vi "Display Hardware Error.vi"(8 "error in (no error)":errorcluster) -> (0 "error out":errorcluster, 3 "Continue?":bool)   [LabVIEW 2020]
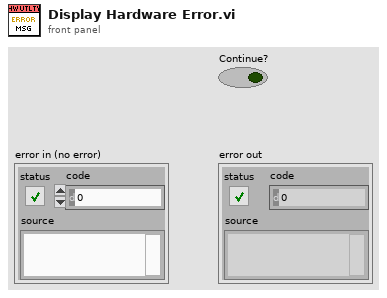
[diagram p1: front panel]
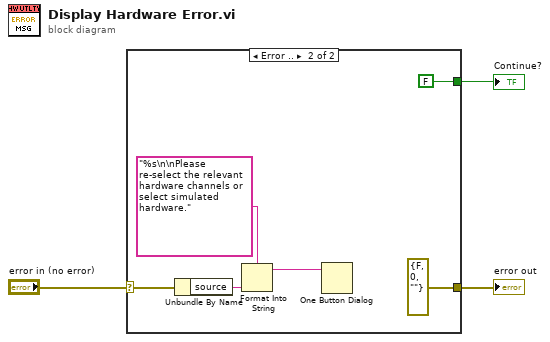
[diagram p0: block diagram]
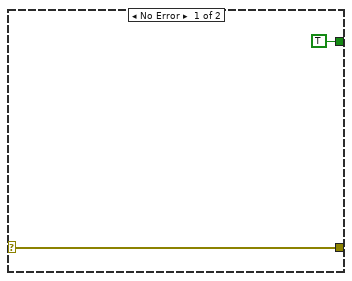
[diagram p2: hidden frame]
diagram:
  n1 = case shown="Error .." "error in (no error)" {
    selector: "error in (no error)" -> [w5 w9]
    tunnel: [w5 errorcluster {"status"=FALSE, "code"=0, "source"=""} ("error IO")] -> w2
    tunnel: [TRUE FALSE] -> w3
    frame No Error {
    }
    frame Error {
      n2 = Unbundle By Name(w9) -> ("source"=w8:string)
      n3 = Format Into String(format string="%s\n\nPlease re-select the relevant hardware channels or select simulated hardware.", w8) -> (resulting string=w7:string)  [unwired: 2 in, 1 out]
      n4 = One Button Dialog(message=w7) -> ()  [unwired: 1 in, 1 out]
    }
  }
  "Continue?" <- w3
  "error out" <- w2
